vi "PanelResizeControl.vi"(5 "TeleopDisplay":refnum<vi>, 6 "MainDashTab":refnum<vi>, 7 "TeleopSubPanel":refnum<vi>, 8 "stopButton":refnum<vi>, 9 "SubPanels":refnum<vi>[](array[refnum]), 10 "TopLevelVI":refnum<vi>, 11 "Window Mode Notifier in":refnum<notifier>) -> ()   [LabVIEW 2015]
uses:
  <vilib>/Utility/miscctls.llb/LVRectTypeDef.ctl
  <vilib>/Utility/miscctls.llb/LVPointTypeDef.ctl
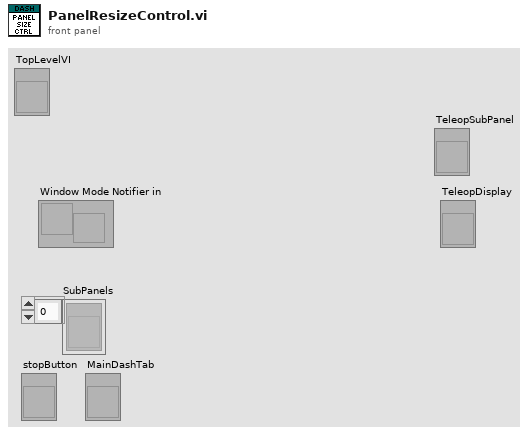
[diagram p1: front panel]
types:
  T1 = typedef "LVRectTypeDef.ctl" = cluster{"Left":i16, "Top":i16, "Right":i16, "Bottom":i16}
  T2 = typedef "LVPointTypeDef.ctl" = cluster{"Horizontal":i16, "Vertical":i16}
  T3 = enum16{"Always On", "Always Off", "Off While Running"}
  T4 = cluster{"TeleopSubPanel":refnum<vi>, "TeleopDisplay":refnum<vi>}
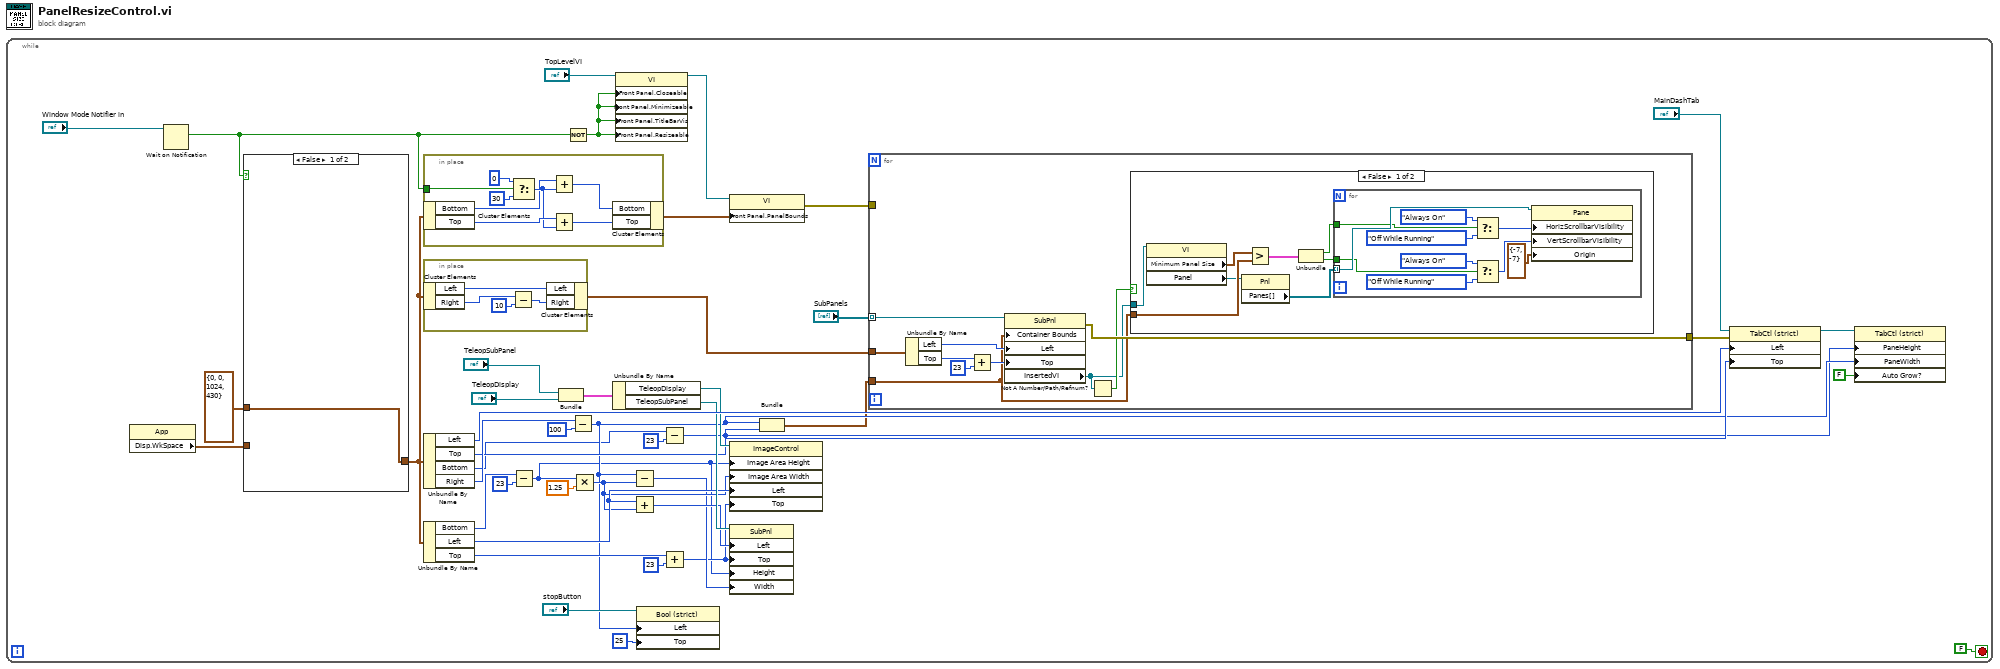
[diagram p0: block diagram]
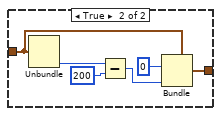
[diagram p3: hidden frame]
diagram:
  n1 = while {
    stop <- FALSE stop-if-true
    n2 = property class="App"() -> ("Disp.WkSpace"=w43:T1)  [unwired: 2 in, 2 out]
    n3 = Wait on Notification(notifier="Window Mode Notifier in") -> (notification=w8:bool)  [unwired: 3 in, 3 out]
    n4 = case shown="False" w8 {
      tunnel: w43 -> [_ w87]
      tunnel: [w85 w88] -> w2
      tunnel: T1 {"Left"=0, "Top"=0, "Right"=1024, "Bottom"=430} ("Front Panel.PanelBounds") -> [w85 _]
      frame False {
      }
      frame True {
        n5 = Unbundle(w87) -> ("Bottom"=w91:i16)  [unwired: 3 out]
        n6 = Subtract(x=w91, y=200) -> (x-y=w89:i32)
        n7 = Bundle(cluster=w87, "Top"=i16 0, "Bottom"=w89) -> (w88:T1)  [unwired: 2 out]
      }
    }
    n8 = in-place {
      in-place-border: w8 -> [w80]
      n9 = in-place-cluster #1(w2) -> ("Bottom"=w77:i16, "Top"=w81:i16)
      n10 = Select(t=i16 0, s=w80, f=i16 30 ("Top")) -> (s? t:f=w79:i16)
      n11 = Add(x=w77, y=w79) -> (x+y=w78:i16)
      n12 = Add(x=w81, y=w79) -> (x+y=w82:i16)
      n13 = in-place-cluster #1("Bottom"=w78, "Top"=w82) -> (w9:T1)
    }
    n14 = in-place {
      n15 = in-place-cluster #2(w2) -> ("Left"=w73:i16, "Right"=w76:i16)
      n16 = Subtract(x=w76, y=i16 10) -> (x-y=w74:i16)
      n17 = in-place-cluster #2("Left"=w73, "Right"=w74) -> (w1:T1)
    }
    n18 = Unbundle By Name(w2) -> ("Left"=w41:i16, "Top"=w17:i16, "Bottom"=w15:i16, "Right"=w40:i16)
    n19 = Unbundle By Name(w2) -> ("Bottom"=w5:i16, "Left"=w33:i16, "Top"=w29:i16)
    n20 = Subtract(x=w5, y=i16 23) -> (x-y=w3:i16)
    n21 = Bundle("TeleopSubPanel"="TeleopSubPanel", "TeleopDisplay"="TeleopDisplay") -> (w36:T4)  [unwired: 1 in]
    n22 = Not(x=w8) -> (.not. x?=w10:bool)
    n23 = Subtract(x=w40, y=i16 100) -> (x-y=w16:i16)
    n24 = Multiply(x=w3, y=1.25) -> (x*y=w31:i32)
    n25 = Unbundle By Name(w36) -> ("TeleopDisplay"=w35:refnum<vi>, "TeleopSubPanel"=w34:refnum<vi>)
    n26 = property class="VI"(reference="TopLevelVI", "Front Panel.Closeable"=w10, "Front Panel.Minimizeable"=w10, "Front Panel.TitleBarVis"=w10, "Front Panel.Resizeable"=w10) -> (reference out=w42:refnum<vi>)  [unwired: 1 in, 1 out]
    n27 = Subtract(x=w16, y=w31) -> (x-y=w30:i32)
    n28 = Add(x=w33, y=w31) -> (x+y=w32:i32)
    n29 = property class="Bool (strict)"(reference="stopButton", "Left"=w16, "Top"=25 ("Position:Top")) -> ()  [unwired: 1 in, 2 out]
    n30 = Subtract(x=w15, y=i16 23) -> (x-y=w14:i16)
    n31 = Add(x=w29, y=i16 23) -> (x+y=w27:i16)
    n32 = property class="VI"(reference=w42, "Front Panel.PanelBounds"=w9) -> (error out=w12:errorcluster)  [unwired: 1 in, 1 out]
    n33 = property class="ImageControl"(reference=w35, "Image Area Height"=w3, "Image Area Width"=w31, "Left"=w33, "Top"=w27) -> ()  [unwired: 1 in, 2 out]
    n34 = property class="SubPnl"(reference=w34, "Left"=w32, "Top"=w27, "Height"=w3, "Width"=w30) -> ()  [unwired: 1 in, 2 out]
    n35 = Bundle(w16, w14) -> (w6:cluster{i16, i16})  [unwired: 1 in]
    n36 = for {
      tunnel: "SubPanels" -> [w54] mode=indexing
      tunnel: w1 -> [w53]
      tunnel: w6 -> [w47]
      tunnel: [w51] -> w18
      tunnel: w12 -> [_]
      n37 = Unbundle By Name(w53) -> ("Left"=w52:i16, "Top"=w50:i16)
      n38 = Add(x=w50, y=i16 23) -> (x+y=w49:i16)
      n39 = property class="SubPnl"(reference=w54, "Container Bounds"=w47, "Left"=w52, "Top"=w49) -> (error out=w51:errorcluster, "InsertedVI"=w45:refnum<vi>)  [unwired: 1 in, 1 out]
      n40 = Not A Number/Path/Refnum?(number/path/refnum=w45) -> (NaN/Path/Refnum?=w46:bool)
      n41 = case shown="False" w46 {
        tunnel: w45 -> [w62 _]
        tunnel: w47 -> [w60 _]
        frame False {
          n42 = property class="VI"(reference=w62) -> ("Minimum Panel Size"=w61:T2, "Panel"=w58:refnum<vi>)  [unwired: 1 in, 2 out]
          n43 = property class="Pnl"(reference=w58) -> ("Panes[]"=w57:refnum<vi>[])  [unwired: 1 in, 2 out]
          n44 = Greater?(x=w61, y=w60) -> (0:w59:cluster{bool, bool})
          n45 = Unbundle(w59) -> (w56:bool, w55:bool)
          n46 = for {
            tunnel: w57 -> [w72] mode=indexing
            tunnel: w56 -> [w68]
            tunnel: w55 -> [w65]
            n47 = Select(t=T3."Always On" ("Vertical Scrollbar Visibility"), s=w68, f=T3."Off While Running") -> (s? t:f=w70:T3)
            n48 = Select(t=T3."Always On" ("Vertical Scrollbar Visibility"), s=w65, f=T3."Off While Running") -> (s? t:f=w64:T3)
            n49 = property class="Pane"(reference=w72, "HorizScrollbarVisibility"=w70, "VertScrollbarVisibility"=w64, "Origin"=T2 {"Horizontal"=-7, "Vertical"=-7}) -> ()  [unwired: 1 in, 2 out]
          }
        }
        frame True {
        }
      }
    }
    n50 = property class="TabCtl (strict)"(reference="MainDashTab", error in=w18, "Left"=w41, "Top"=w17) -> (reference out=w7:refnum<vi>)  [unwired: 1 out]
    n51 = property class="TabCtl (strict)"(reference=w7, "PaneHeight"=w14, "PaneWidth"=w16, "Auto Grow?"=FALSE) -> ()  [unwired: 1 in, 2 out]
  }
